vi "Update Target Deployment Status.vi"(6 "Add Timestamp?":bool, 7 "Column":i32=2, 8 "error out":errorcluster, 9 "Target Index":i32, 10 "Message":string="Successfully deployed.", 11 "Targets Deployment Status":string[][](array[string])) -> (3 "Targets Deployment Status":string[][](array[string]))   [LabVIEW 2020]
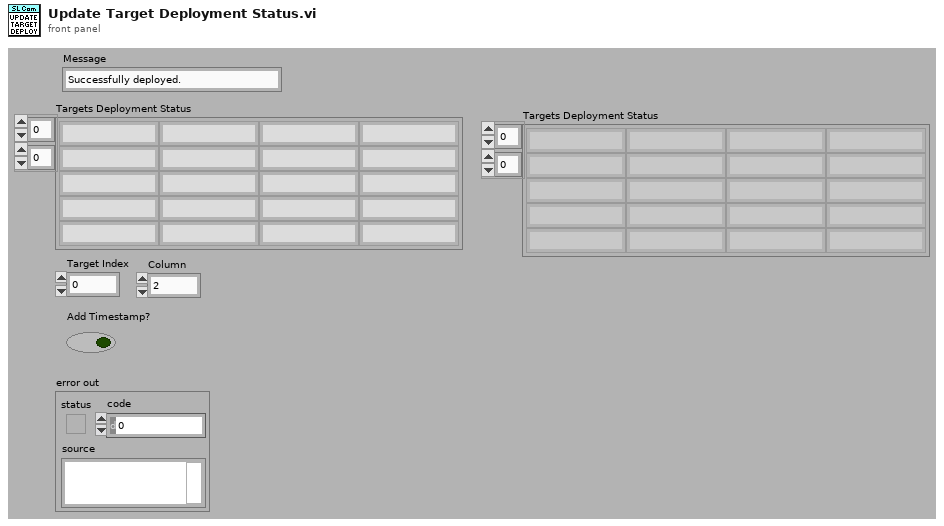
[diagram p1: front panel]
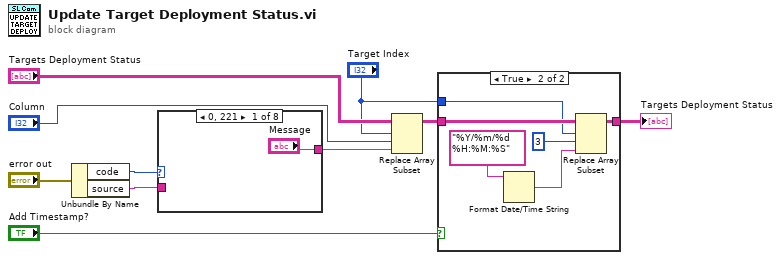
[diagram p0: block diagram]
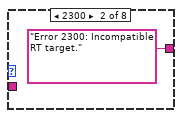
[diagram p3: hidden frame]
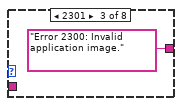
[diagram p4: hidden frame]
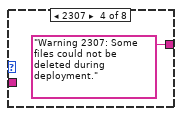
[diagram p5: hidden frame]
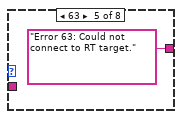
[diagram p6: hidden frame]
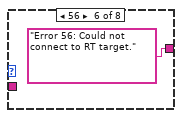
[diagram p7: hidden frame]
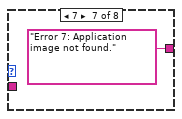
[diagram p8: hidden frame]
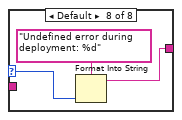
[diagram p9: hidden frame]
diagram:
  n1 = Unbundle By Name("error out") -> ("code"=w5:i32, "source"=w6:string)
  n2 = case shown="0, 221" w5 {
    selector: w5 -> [_ _ _ _ _ _ _ w18]
    tunnel: ["Message" "Error 2300: Incompatible RT target." "Error 2300: Invalid application image." "Warning 2307: Some files could not be deleted during deployment." ("Message") "Error 63: Could not connect to RT target." "Error 56: Could not connect to RT target." "Error 7: Application image not found." w20] -> w8
    tunnel: w6 -> [_ _ _ _ _ _ _ _]
    frame 0, 221 {
    }
    frame 2300 {
    }
    frame 2301 {
    }
    frame 2307 {
    }
    frame 63 {
    }
    frame 56 {
    }
    frame 7 {
    }
    frame Default {
      n3 = Format Into String(format string="Undefined error during deployment: %d", w18) -> (resulting string=w20:string)  [unwired: 2 in, 1 out]
    }
  }
  n4 = Replace Array Subset(array="Targets Deployment Status", new element=w8, index (row)="Target Index", index (col)="Column") -> (w4:string[][])
  n5 = case shown="True" "Add Timestamp?" {
    tunnel: w4 -> [w21 w27]
    tunnel: "Target Index" -> [_ w23]
    tunnel: [w21 w22] -> w2
    frame False {
    }
    frame True {
      n6 = Format Date/Time String(time format string (%c)="%Y/%m/%d %H:%M:%S") -> (date/time string=w25:string)  [unwired: 2 out]
      n7 = Replace Array Subset(array=w27, new element=w25, index (row)=w23, index (col)=3 ("disabled index (col)")) -> (w22:string[][])
    }
  }
  "Targets Deployment Status" <- w2
